vi "SetFreqRatio.vi"(8 "错误输入（无错误）":errorcluster, 10 "滤波模式索引值":u16) -> (0 "错误输出":errorcluster)   [LabVIEW 2014]
uses:
  X86Dll/ZXUTConfigMgr.dll
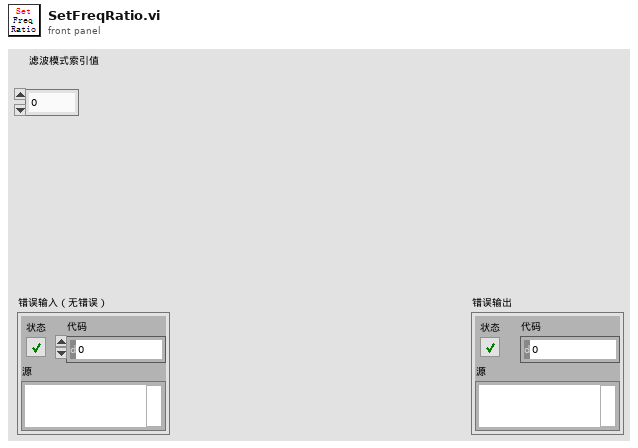
[diagram p1: front panel]
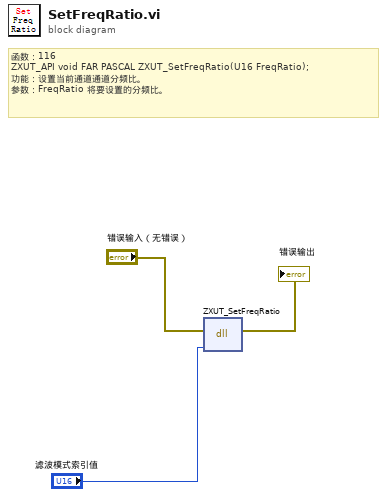
[diagram p0: block diagram]
diagram:
  # "函数：116\nZXUT_API void\tFAR PASCAL ZXUT_SetFreqRatio(U16 FreqRatio);\n功能：设置当前通道通道分频比。\n参数：FreqRatio 将要设置的分频比。"
  n1 = dll-call lib="D:/Software/Utrasonic on-line monitoring/X86Dll/ZXUTConfigMgr.dll" fn="ZXUT_SetFreqRatio"(error in="错误输入（无错误）", "SetFreqRatio"="滤波模式索引值") -> (error out=→"错误输出":errorcluster)  [unwired: 4 in, 1 out]
